vi "Update Mode.vi"(6 "Refresh Channels? (T)":bool=TRUE, 7 "Go to first chan?":bool=TRUE, 8 "error in (no error)":errorcluster, 9 "SD Control Refs in":T2, 10 "SD Module in":refnum<class "SD Module.lvclass">, 11 "Node Ptr In":T1 format="%.0x") -> (0 "error out":errorcluster, 1 "SD Control Refs out":T2, 2 "SD Module out":refnum<class "SD Module.lvclass">, 3 "Node Ptr Out":T1 format="%.0x")   [LabVIEW 2020, in "Modules.lvlib" / "SD Module.lvclass"]
uses:
  SD Module.lvclass
  C:/Users/nitest/Desktop/Git 2020/niveristand-scan-engine-module-libraries/Source/RSI Module/RSI Module.lvclass
  Type Defs/SD Control Refs.ctl
  Type Defs/Main Control Refs.ctl
  Type Defs/Counter Control Refs.ctl
  Type Defs/CDO Control Refs.ctl
  Type Defs/PWM Control Refs.ctl
  Type Defs/Quadrature Control Refs.ctl
  <vilib>/NI VeriStand/Custom Device API/Custom Device Item Ref.ctl
  SD Module.lvclass/SD Module.ctl
  RSI Module/Channel Type.ctl
  RSI Module/Channels.ctl
  <vilib>/NI VeriStand/Custom Device API/Custom Device Channel Type.ctl
  Type Defs/_nicrio_ChannelsControl.ctl
  <vilib>/NI VeriStand/Custom Device API/Custom Device API.lvlib
  RSI Module/RSI Module.lvclass
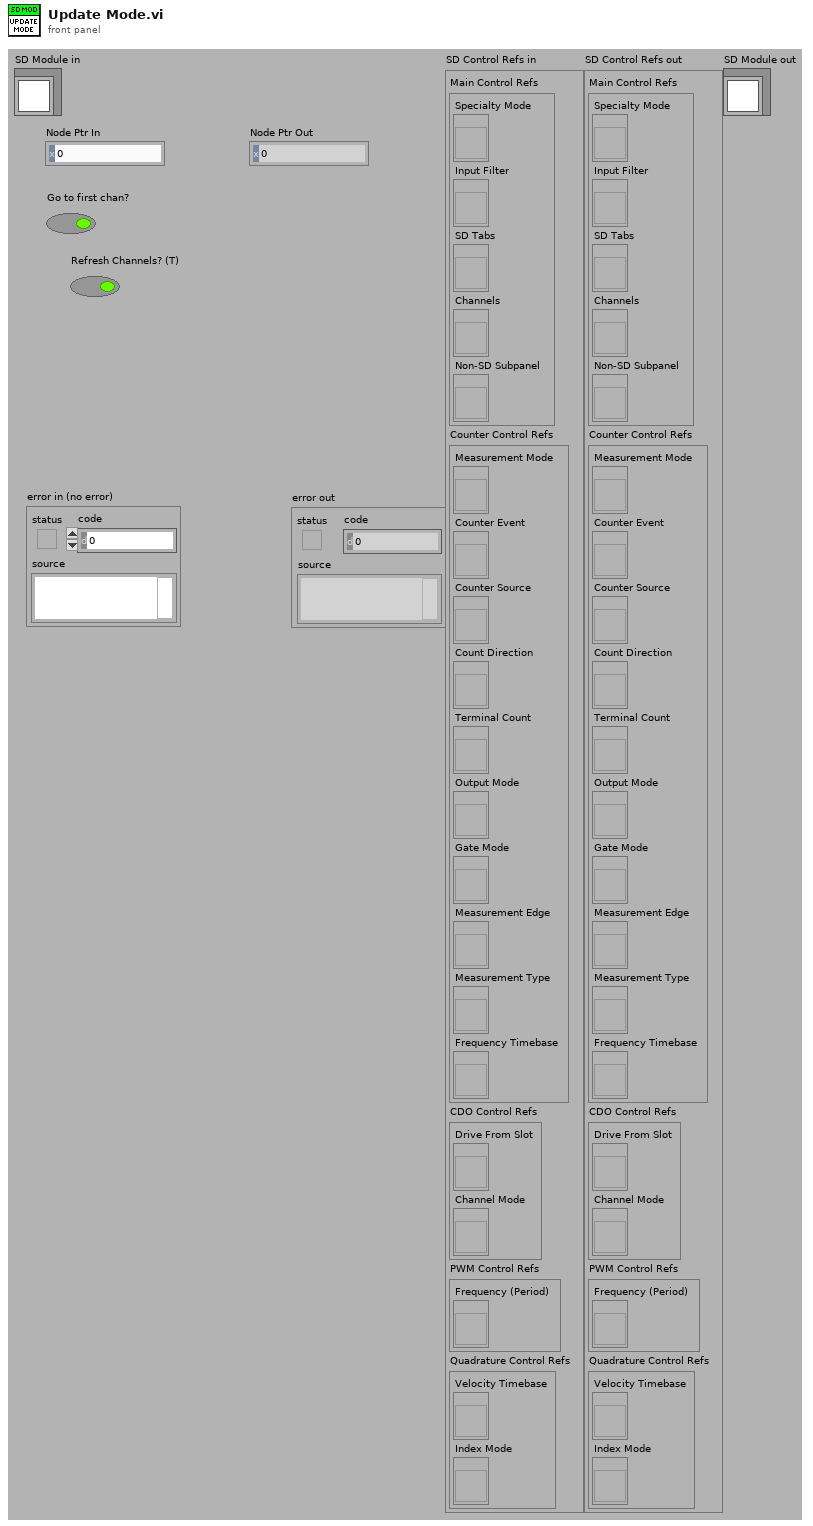
[diagram p1: front panel]
types:
  T1 = typedef "Custom Device API.lvlib/Custom Device Item Ref.ctl" = u64
  T2 = typedef "Modules.lvlib/SD Module.lvclass/SD Control Refs.ctl" = cluster{"Main Control Refs":T3, "Counter Control Refs":T4, "CDO Control Refs":T5, "PWM Control Refs":T6, "Quadrature Control Refs":T7}
  T3 = typedef "Modules.lvlib/SD Module.lvclass/Main Control Refs.ctl" = cluster{"Specialty Mode":refnum<vi>, "Input Filter":refnum<vi>, "SD Tabs":refnum<vi>, "Channels":refnum<vi>, "Non-SD Subpanel":refnum<vi>}
  T4 = typedef "Modules.lvlib/SD Module.lvclass/Counter Control Refs.ctl" = cluster{"Measurement Mode":refnum<vi>, "Counter Event":refnum<vi>, "Counter Source":refnum<vi>, "Count Direction":refnum<vi>, "Terminal Count":refnum<vi>, "Output Mode":refnum<vi>, "Gate Mode":refnum<vi>, "Measurement Edge":refnum<vi>, "Measurement Type":refnum<vi>, "Frequency Timebase":refnum<vi>}
  T5 = typedef "Modules.lvlib/SD Module.lvclass/CDO Control Refs.ctl" = cluster{"Drive From Slot":refnum<vi>, "Channel Mode":refnum<vi>}
  T6 = typedef "Modules.lvlib/SD Module.lvclass/PWM Control Refs.ctl" = cluster{"Frequency (Period)":refnum<vi>}
  T7 = typedef "Modules.lvlib/SD Module.lvclass/Quadrature Control Refs.ctl" = cluster{"Velocity Timebase":refnum<vi>, "Index Mode":refnum<vi>}
  T8 = typedef "Custom Device API.lvlib/Custom Device Channel Type.ctl" = enum16{"Input", "Output"}
  T9 = typedef "Modules.lvlib/RSI Module.lvclass/Channels.ctl" = cluster{"# Input Channels":i32, "# Output Channels":i32, "Channel Type":T10, "Units":string}
  T10 = typedef "Modules.lvlib/RSI Module.lvclass/Channel Type.ctl" = enum16{"Analog", "Digital"}
  T11 = typedef "Modules.lvlib/SD Module.lvclass/_nicrio_ChannelsControl.ctl" = i32
  T12 = typedef "Modules.lvlib/SD Module.lvclass/Counter Channel.ctl" = cluster{"Measurement Mode":u32, "Count Edges":T13, "Period Measurement":T14, "Pulse Width Measurement":T15, "Frequency Measurement":T16}
  T13 = typedef "Modules.lvlib/SD Module.lvclass/Count Edges.ctl" = cluster{"Counter Event":u32, "Counter Source":u32, "Counter Direction":u32, "Terminal Count":u32, "Output Mode":u32, "Gate Mode":u32}
  T14 = typedef "Modules.lvlib/SD Module.lvclass/Period Measurement.ctl" = cluster{"Measurement Edge":u32}
  T15 = typedef "Modules.lvlib/SD Module.lvclass/Pulse Width Measurement.ctl" = cluster{"Measurement Type":u32}
  T16 = typedef "Modules.lvlib/SD Module.lvclass/Frequency Measurement.ctl" = cluster{"Measurement Edge":u32, "Measurement Timebase":u32}
  T17 = typedef "Modules.lvlib/SD Module.lvclass/CDO Channel.ctl" = cluster{"Counter driven enabled":bool}
  T18 = typedef "Modules.lvlib/SD Module.lvclass/PWM Channel.ctl" = cluster{"PWM frequency":u32}
  T19 = typedef "Modules.lvlib/SD Module.lvclass/Quadrature Channel.ctl" = cluster{"Timebase":u32, "Index Mode":u32}
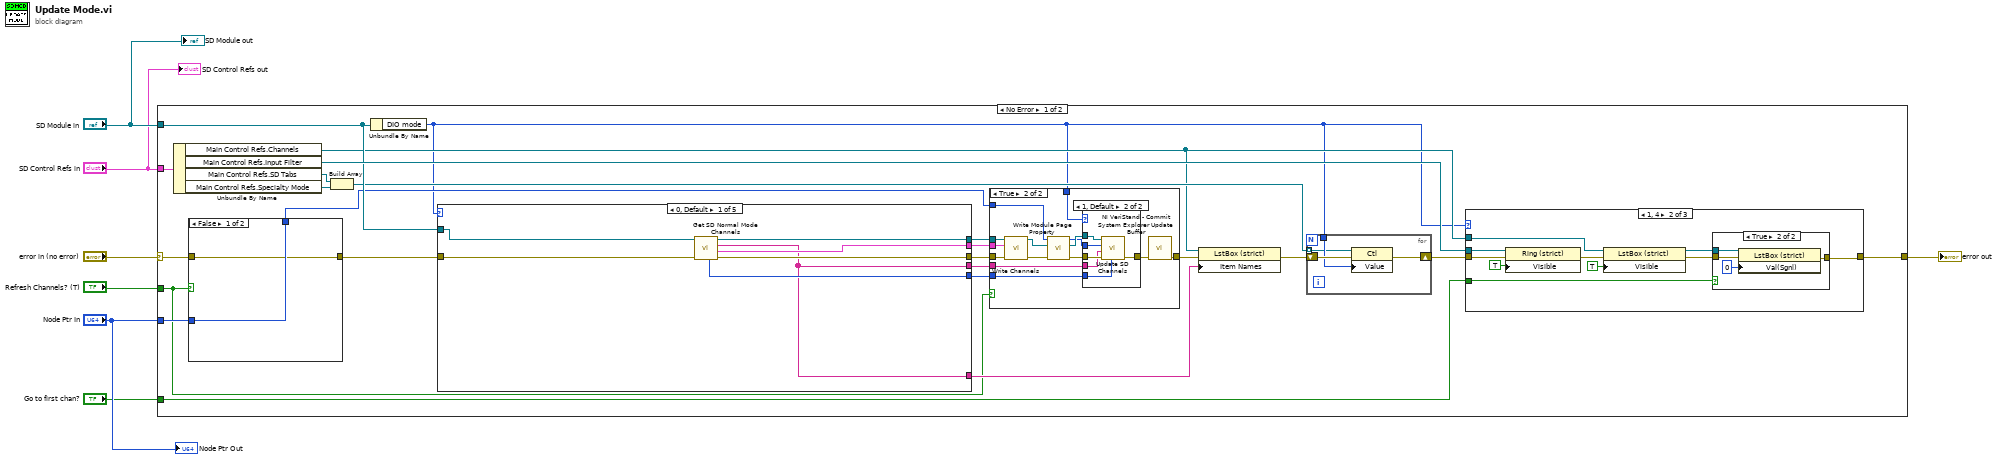
[diagram p0: block diagram]
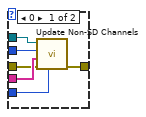
[diagram p3: hidden frame]
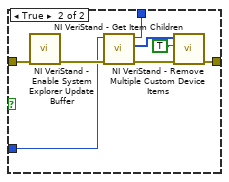
[diagram p4: hidden frame]
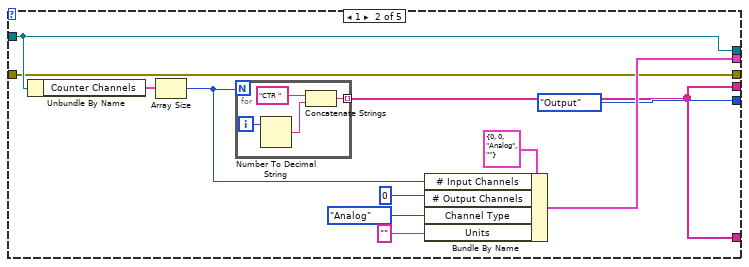
[diagram p5: hidden frame]
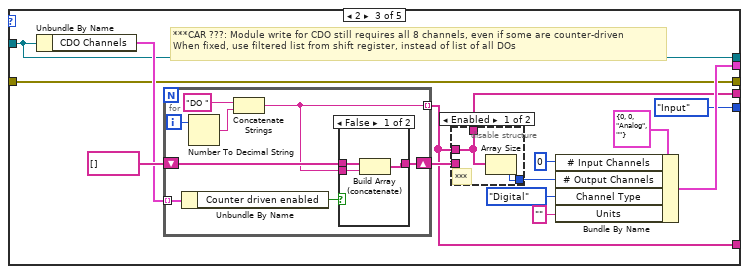
[diagram p6: hidden frame]
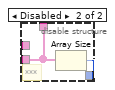
[diagram p7: hidden frame]
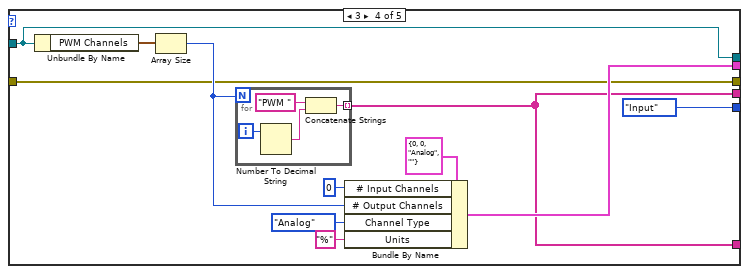
[diagram p9: hidden frame]
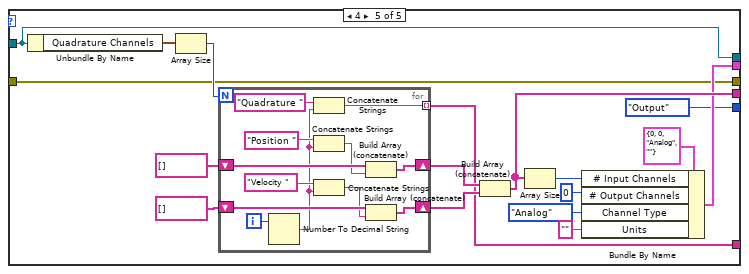
[diagram p10: hidden frame]
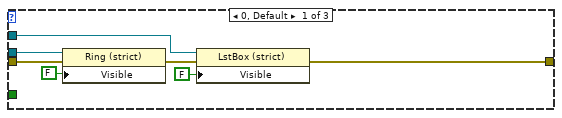
[diagram p11: hidden frame]
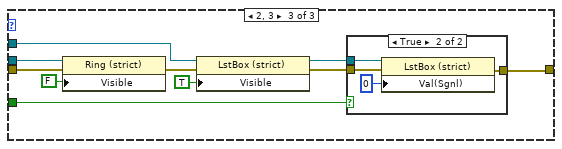
[diagram p13: hidden frame]
diagram:
  n1 = case shown="No Error" "error in (no error)" {
    selector: "error in (no error)" -> [w24 w206]
    tunnel: [w29 w206] -> w5
    tunnel: "SD Control Refs in" -> [w25 _]
    tunnel: "SD Module in" -> [w30 _]
    tunnel: "Node Ptr In" -> [w23 _]
    tunnel: "Go to first chan?" -> [w13 _]
    tunnel: "Refresh Channels? (T)" -> [w8 _]
    frame No Error {
      n2 = Unbundle By Name(w25) -> ("Main Control Refs.Channels"=w15:refnum<vi>, "Main Control Refs.Input Filter"=w31:refnum<vi>, "Main Control Refs.SD Tabs"=w28:refnum<vi>, "Main Control Refs.Specialty Mode"=w27:refnum<vi>)
      n3 = case shown="False" w8 {
        tunnel: w24 -> [w59 w67]
        tunnel: w23 -> [w60 w63]
        tunnel: [w59 w62] -> w18
        tunnel: [w60 w61] -> w12
        frame False {
        }
        frame True {
          n4 = call <vilib>:"NI VeriStand - Enable System Explorer Update Buffer.vi"("error in (no error)"=w67) -> ("error out"=w66:errorcluster)  [unwired: 10 in]
          n5 = call <vilib>:"NI VeriStand - Get Item Children.vi"("error in (no error)"=w66, "Item Ref in"=w63) -> ("error out"=w64:errorcluster, "Child Refs"=w65:T1[], "Item Ref out"=w61:T1)  [unwired: 6 in, 1 out]
          n6 = call <vilib>:"NI VeriStand - Remove Multiple Custom Device Items.vi"("error in (no error)"=w64, "Force Delete (F)"=TRUE, "Item Refs in"=w65) -> ("error out"=w62:errorcluster)  [unwired: 7 in, 1 out]
        }
      }
      n7 = Build Array(w28, w27) -> (w26:refnum<vi>[])
      n8 = Unbundle By Name(w30) -> ("DIO mode"=w9:u32)
      n9 = case shown="0, Default" w9 {
        tunnel: [w78 w81 w98 w125 w140] -> w22
        tunnel: w18 -> [w79 w81 w98 w125 w140]
        tunnel: w30 -> [w77 w82 w99 w127 w142]
        tunnel: [w73 w80 w97 w126 w145] -> w11
        tunnel: [w76 w84 w101 w129 w144] -> w20
        tunnel: [w75 w82 w99 w127 w142] -> w21
        tunnel: [w74 Custom_Device_Channel_Type."Output" ("Type") Custom_Device_Channel_Type."Input" ("Type") Custom_Device_Channel_Type."Input" ("Type") Custom_Device_Channel_Type."Output" ("Type")] -> w10
        tunnel: [w73 w80 w95 w126 w141] -> w14
        frame 0, Default {
          n10 = call-dynamic "Get SD Normal Mode Channels.vi"("error in (no error)"=w79, "SD Module in"=w77) -> ("error out"=w78:errorcluster, "Channels"=w76:T9, "Channel Names"=w73:string[], "SD Module out"=w75:refnum<class "SD Module.lvclass">, "Type"=w74:T8)  [unwired: 5 in]
        }
        frame 1 {
          n11 = Unbundle By Name(w82) -> ("Counter Channels"=w90:T12[])
          n12 = Array Size(array=w90) -> (size(s)=w85:i32)
          n13 = for {
            N: w85 -> [_]
            tunnel: [w91] -> w80 mode=indexing
            i -> [w94]
            n14 = Number To Decimal String(number=w94) -> (decimal integer string=w92:string)  [unwired: 1 in]
            n15 = Concatenate Strings("CTR ", w92) -> (w91:string)
          }
          n16 = Bundle By Name(cluster=T9 {"# Input Channels"=0, "# Output Channels"=0, "Channel Type"=enum."Analog", "Units"=""} ("Channels"), "# Input Channels"=w85, "# Output Channels"=0, "Channel Type"=Channel_Type."Analog", "Units"="") -> (w84:T9)
        }
        frame 2 {
          # "***CAR ???: Module write for CDO still requires all 8 channels, even if some are counter-driven\nWhen fixed, use filtered list from shift register, instead of list of all DOs"
          n17 = Unbundle By Name(w99) -> ("CDO Channels"=w103:T17[])
          n18 = for {
            tunnel: [w113] -> w95 mode=indexing
            shift-right: [w114] -> w96
            shift-left: string[] [] -> [w115]
            tunnel: w103 -> [w117] mode=indexing
            i -> [w120]
            n19 = Unbundle By Name(w117) -> ("Counter driven enabled"=w116:bool)
            n20 = Number To Decimal String(number=w120) -> (decimal integer string=w118:string)  [unwired: 1 in]
            n21 = Concatenate Strings("DO ", w118) -> (w113:string)
            n22 = case shown="False" w116 {
              tunnel: w115 -> [w123 w124]
              tunnel: w113 -> [w122 _]
              tunnel: [w121 w124] -> w114
              frame False {
                n23 = Build Array (concatenate)(w123, w122) -> (w121:string[])
              }
              frame True {
              }
            }
          }
          n24 = disable-structure shown="Enabled" {
            disable-tunnel: [w110 w112] -> w102
            disable-tunnel: [w109 w111] -> w97
            disable-tunnel: w96 -> [_ w111]
            disable-tunnel: w95 -> [w109 _]
            frame Enabled {
              # "***"
              n25 = Array Size(array=w109) -> (size(s)=w110:i32)
            }
            frame Disabled {
              # "***"
              n26 = Array Size(array=w111) -> (size(s)=w112:i32)
            }
          }
          n27 = Bundle By Name(cluster=T9 {"# Input Channels"=0, "# Output Channels"=0, "Channel Type"=enum."Analog", "Units"=""} ("Channels"), "# Input Channels"=0, "# Output Channels"=w102, "Channel Type"=Channel_Type."Digital", "Units"="") -> (w101:T9)
        }
        frame 3 {
          n28 = Unbundle By Name(w127) -> ("PWM Channels"=w135:T18[])
          n29 = Array Size(array=w135) -> (size(s)=w130:i32)
          n30 = for {
            N: w130 -> [_]
            tunnel: [w136] -> w126 mode=indexing
            i -> [w139]
            n31 = Number To Decimal String(number=w139) -> (decimal integer string=w137:string)  [unwired: 1 in]
            n32 = Concatenate Strings("PWM ", w137) -> (w136:string)
          }
          n33 = Bundle By Name(cluster=T9 {"# Input Channels"=0, "# Output Channels"=0, "Channel Type"=enum."Analog", "Units"=""} ("Channels"), "# Input Channels"=0, "# Output Channels"=w130, "Channel Type"=Channel_Type."Analog", "Units"="%") -> (w129:T9)
        }
        frame 4 {
          n34 = Unbundle By Name(w142) -> ("Quadrature Channels"=w155:T19[])
          n35 = Array Size(array=w155) -> (size(s)=w156:i32)
          n36 = for {
            N: w156 -> [_]
            tunnel: [w166] -> w141 mode=indexing
            shift-right: [w158] -> w148
            shift-left: string[] [] -> [w165]
            shift-right: [w157] -> w147
            shift-left: string[] [] -> [w164]
            i -> [w168]
            n37 = Number To Decimal String(number=w168) -> (decimal integer string=w160:string)  [unwired: 1 in]
            n38 = Concatenate Strings("Quadrature ", w160) -> (w166:string)
            n39 = Concatenate Strings("Position ", w160) -> (w162:string)
            n40 = Concatenate Strings("Velocity ", w160) -> (w159:string)
            n41 = Build Array (concatenate)(w165, w162) -> (w158:string[])
            n42 = Build Array (concatenate)(w164, w159) -> (w157:string[])
          }
          n43 = Build Array (concatenate)(w148, w147) -> (w145:string[])
          n44 = Array Size(array=w145) -> (size(s)=w146:i32)
          n45 = Bundle By Name(cluster=T9 {"# Input Channels"=0, "# Output Channels"=0, "Channel Type"=enum."Analog", "Units"=""} ("Channels"), "# Input Channels"=w146, "# Output Channels"=0, "Channel Type"=Channel_Type."Analog", "Units"="") -> (w144:T9)
        }
      }
      n46 = case shown="True" w8 {
        tunnel: w22 -> [w32 w46]
        tunnel: w21 -> [_ w45]
        tunnel: w20 -> [_ w44]
        tunnel: [w32 w43] -> w17
        tunnel: w12 -> [_ w41]
        tunnel: w11 -> [_ w37]
        tunnel: w10 -> [_ w36]
        tunnel: w9 -> [_ w33]
        frame False {
        }
        frame True {
          n47 = call "Write Channels.vi"("error in (no error)"=w46, "Channels"=w44, "RSI Module in"=w45) -> ("error out"=w42:errorcluster, "RSI Module out"=w40:refnum<class "SD Module.lvclass">)  [unwired: 7 in]
          n48 = call "Write Module Page Property.vi"("error in (no error)"=w42, "RSI Module"=w40, "Node Ptr In"=w41) -> ("error out"=w35:errorcluster, "RSI Module out"=w39:refnum<class "SD Module.lvclass">, "Node Ptr Out"=w38:T1)  [unwired: 6 in]
          n49 = case shown="1, Default" w33 {
            tunnel: w39 -> [w52 w55]
            tunnel: w38 -> [w51 w54]
            tunnel: w37 -> [w50 w53]
            tunnel: w36 -> [w49 w56]
            tunnel: w35 -> [w48 w58]
            tunnel: [w47 w57] -> w34
            frame 0 {
              n50 = call-dynamic "Update Non-SD Channels.vi"("Type"=w49, "error in (no error)"=w48, "Channel Names"=w50, "Node Ptr In"=w51, "SD Module in"=w52) -> ("error out"=w47:errorcluster)  [unwired: 4 in, 2 out]
            }
            frame 1, Default {
              n51 = call "Update SD Channels.vi"("Type"=w56, "error in (no error)"=w58, "Channel Names"=w53, "Node Ptr In"=w54, "SD Module in"=w55) -> ("error out"=w57:errorcluster)  [unwired: 4 in, 2 out]
            }
          }
          n52 = call <vilib>:"NI VeriStand - Commit System Explorer Update Buffer.vi"("error in (no error)"=w34) -> ("error out"=w43:errorcluster)  [unwired: 10 in]
        }
      }
      n53 = property class="LstBox (strict)"(reference=w15, error in=w17, "Item Names"=w14) -> (error out=w16:errorcluster)  [unwired: 1 out]
      n54 = for {
        tunnel: w9 -> [w70]
        shift-right: [w71] -> w19
        shift-left: w16 -> [w72]
        tunnel: w26 -> [w69] mode=indexing
        n55 = property class="Ctl"(reference=w69, error in=w72, "Value"=w70) -> (error out=w71:errorcluster)  [unwired: 1 out]
      }
      n56 = case shown="1, 4" w9 {
        tunnel: [w172 w176 w191] -> w29
        tunnel: w19 -> [w171 w182 w197]
        tunnel: w31 -> [w170 w181 w196]
        tunnel: w15 -> [w169 w180 w195]
        tunnel: w13 -> [_ w177 w192]
        frame 0, Default {
          n57 = property class="Ring (strict)"(reference=w170, error in=w171, "Visible"=FALSE) -> (error out=w175:errorcluster)  [unwired: 1 out]
          n58 = property class="LstBox (strict)"(reference=w169, error in=w175, "Visible"=FALSE) -> (error out=w172:errorcluster)  [unwired: 1 out]
        }
        frame 1, 4 {
          n59 = property class="Ring (strict)"(reference=w181, error in=w182, "Visible"=TRUE) -> (error out=w185:errorcluster)  [unwired: 1 out]
          n60 = property class="LstBox (strict)"(reference=w180, error in=w185, "Visible"=TRUE) -> (reference out=w179:refnum<vi>, error out=w178:errorcluster)
          n61 = case shown="True" w177 {
            tunnel: w179 -> [_ w190]
            tunnel: w178 -> [w186 w189]
            tunnel: [w186 w187] -> w176
            frame False {
            }
            frame True {
              n62 = property class="LstBox (strict)"(reference=w190, error in=w189, "Val(Sgnl)"=T11 0 ("Value (Signaling)")) -> (error out=w187:errorcluster)  [unwired: 1 out]
            }
          }
        }
        frame 2, 3 {
          n63 = property class="Ring (strict)"(reference=w196, error in=w197, "Visible"=FALSE) -> (error out=w200:errorcluster)  [unwired: 1 out]
          n64 = property class="LstBox (strict)"(reference=w195, error in=w200, "Visible"=TRUE) -> (reference out=w193:refnum<vi>, error out=w194:errorcluster)
          n65 = case shown="True" w192 {
            tunnel: w193 -> [_ w205]
            tunnel: w194 -> [w201 w204]
            tunnel: [w201 w202] -> w191
            frame False {
            }
            frame True {
              n66 = property class="LstBox (strict)"(reference=w205, error in=w204, "Val(Sgnl)"=T11 0 ("Value (Signaling)")) -> (error out=w202:errorcluster)  [unwired: 1 out]
            }
          }
        }
      }
    }
    frame Error {
    }
  }
  "error out" <- w5
  "SD Control Refs out" <- "SD Control Refs in"
  "SD Module out" <- "SD Module in"
  "Node Ptr Out" <- "Node Ptr In"
